vi "TagRead.vi"(7 "LabVIEW Web Service Request":refnum<class "Web Request.lvclass">, 10 "type":T1, 11 "tagName":T2) -> ()   [LabVIEW 2013]
uses:
  <vilib>/wsapi/Web Request.lvclass
  <vilib>/NI/TagWebClient/API/String Controls/tagName.ctl
  <vilib>/NI/TagWebClient/API/String Controls/type.ctl
  <vilib>/NI/Tag Bus/tag/Data Type.ctl
  <vilib>/NI/Tag Bus/table/data table.ctl
  <vilib>/NI/TagWebClient/API/JSON Formats/TagRead Response.ctl
  <vilib>/NI/TagWebClient/API/String Controls/value.ctl
  <vilib>/NI/Tag Bus/dictionary/data dictionary.lvclass
  <vilib>/NI/Tag Bus/tag/tag descriptor.lvclass
  <vilib>/NI/Tag Bus/table/data table.lvlib
  <vilib>/NI/TagWebClient/API/tagweb client API.lvlib
panel:
  out "Response String":string
  # "Use the Web Service Request input terminal to call the VIs on the Web Services palette. Do not remove it from the connector pane unless you don't need access to the palette."
  # "Each additional control wired to the connector pane will be available as an input in the URL. To include an indicator in terminal-mode output (the default setting), it must also be wired to the connector pane."
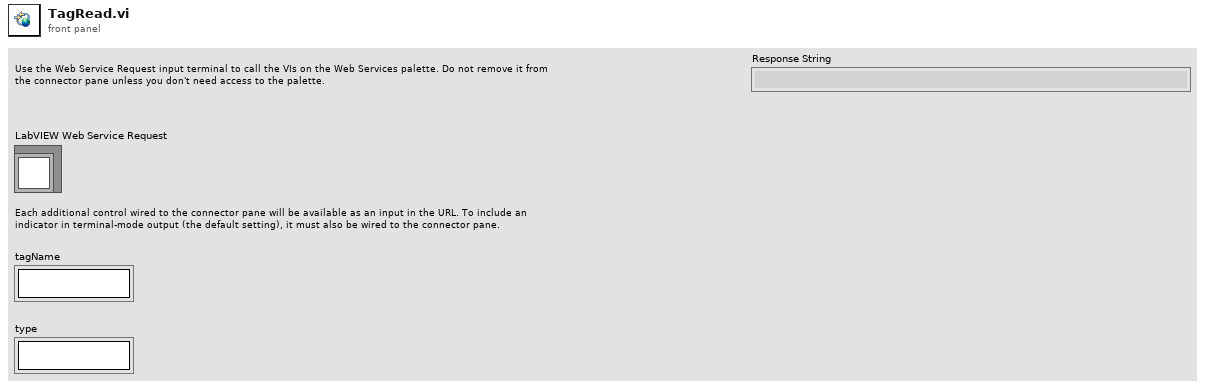
[diagram p1: front panel]
types:
  T1 = typedef "tagweb client API.lvlib/type.ctl" = string
  T2 = typedef "tagweb client API.lvlib/tagName.ctl" = string
  T3 = typedef "tag bus.lvlib/tag descriptor.lvclass/Data Type.ctl" = enum16{"Double", "Single", "I64", "I32", "I16", "I8", "U64", "U32", "U16", "U8", "Boolean", "String", "Array of Double", "Array of Single", "Array of I64", "Array of I32", "Array of I16", "Array of I8", "Array of U64", "Array of U32", "Array of U16", "Array of U8", "Array of Boolean", "Array of String"}
  T4 = typedef "tag bus.lvlib/data table.lvlib/data table.ctl" = cluster{"Double":dbl[], "Single":sgl[], "I64":i64[], "I32":i32[], "I16":i16[], "I8":i8[], "U64":u64[], "U32":u32[], "U16":u16[], "U8":u8[], "Boolean":bool[], "String":string[], "Array of Double":cluster{"DBL Array":dbl[]}[], "Array of Single":cluster{"SGL Array":sgl[]}[], "Array of I64":cluster{"I64 Array":i64[]}[], "Array of I32":cluster{"I32 Array":i32[]}[], "Array of I16":cluster{"I16 Array":i16[]}[], "Array of I8":cluster{"I8 Array":i8[]}[], "Array of U64":cluster{"U64 Array":u64[]}[], "Array of U32":cluster{"U32 Array":u32[]}[], "Array of U16":cluster{"U16 Array":u16[]}[], "Array of U8":cluster{"U8 Array":u8[]}[], "Array of Boolean":cluster{"Boolean Array":bool[]}[], "Array of String":cluster{"String Array":string[]}[]}
  T5 = typedef "tagweb client API.lvlib/TagRead Response.ctl" = cluster{"value":T6}
  T6 = typedef "tagweb client API.lvlib/value.ctl" = string
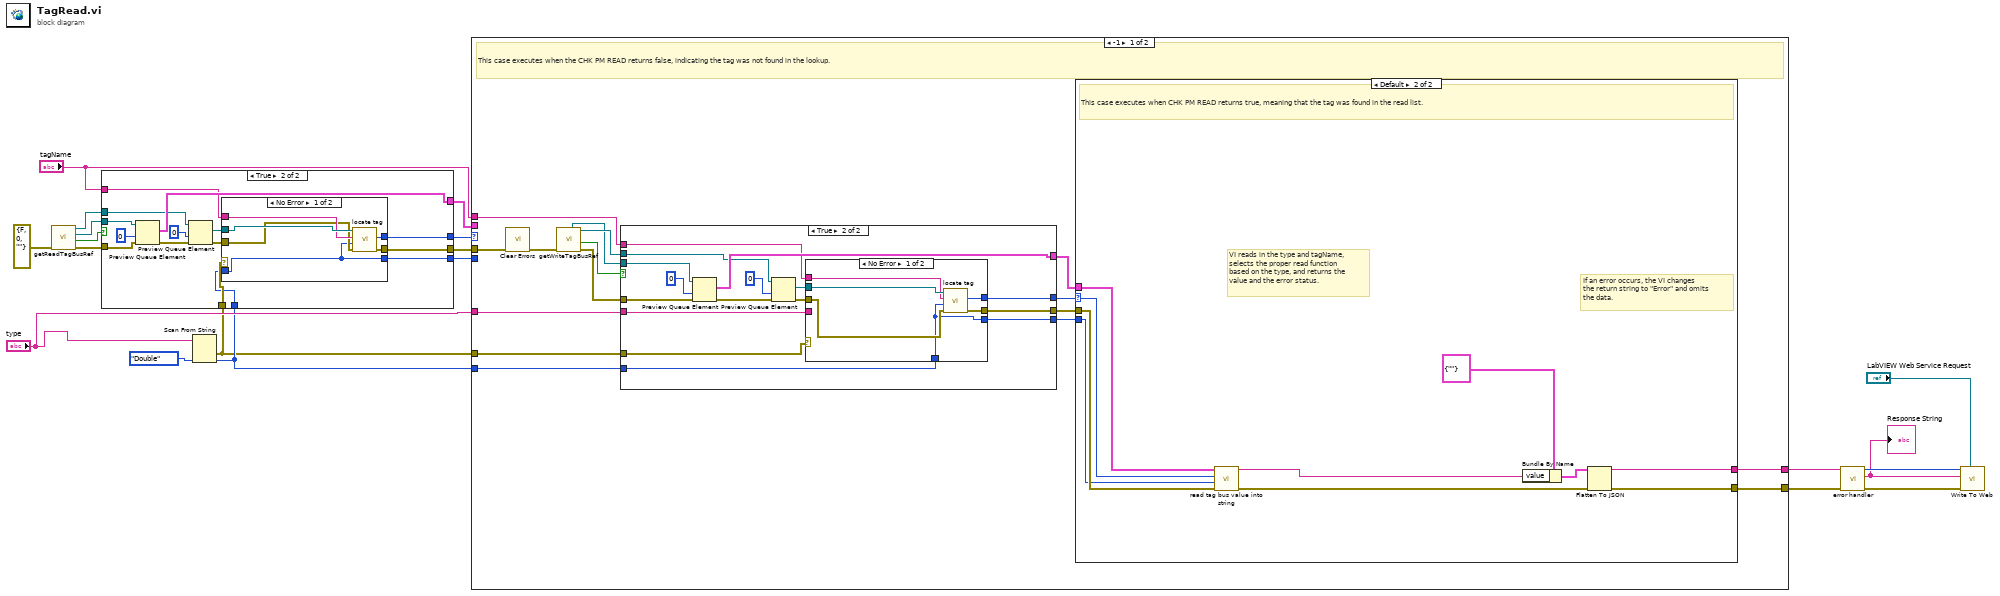
[diagram p0: block diagram]
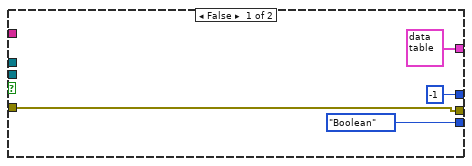
[diagram p2: hidden frame]
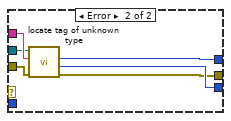
[diagram p3: hidden frame]
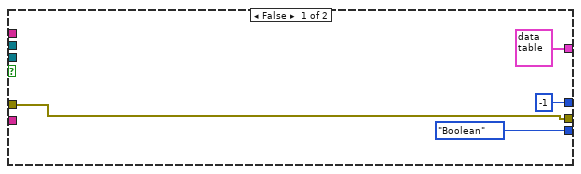
[diagram p4: hidden frame]
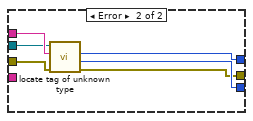
[diagram p5: hidden frame]
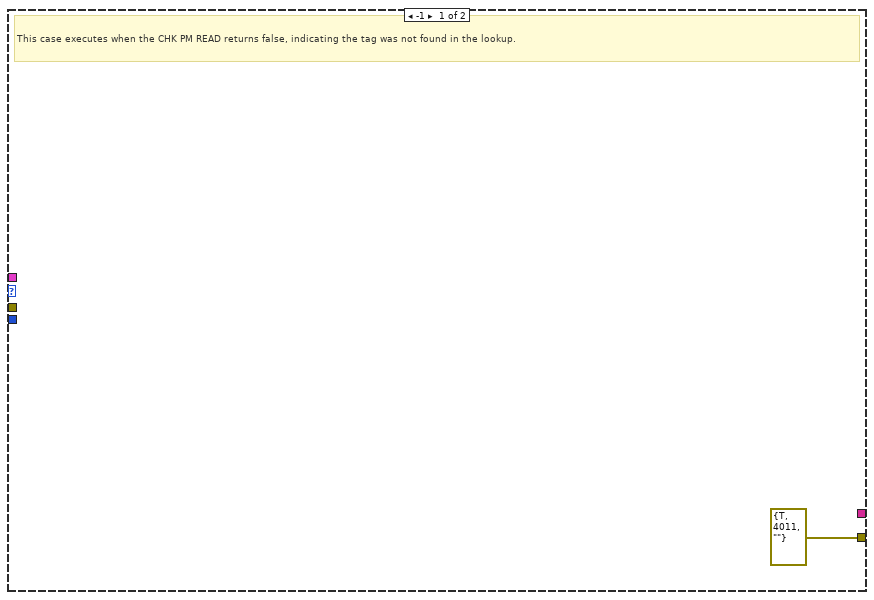
[diagram p6: hidden frame]
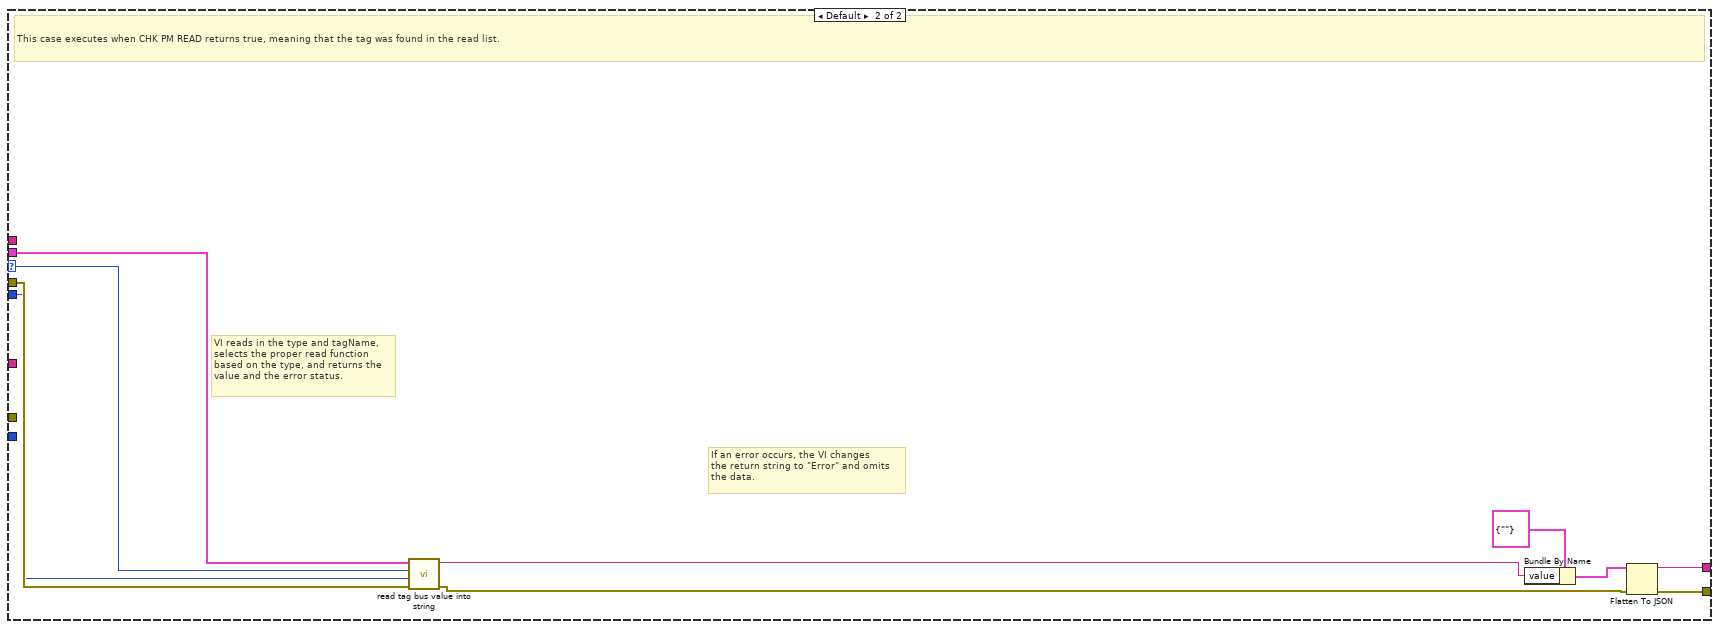
[diagram p7: hidden frame]
diagram:
  n1 = call "getReadTagBusRef.vi"("error in (no error)"=errorcluster {"status"=FALSE, "code"=0, "source"=""}) -> ("error out"=w13:errorcluster, "valid references"=w12:bool, "read data table"=w11:refnum<queue>, "read data dictionary"=w9:refnum<queue>)  [unwired: 7 in]
  n2 = Scan From String(input string="type", default 1=Data_Type."Double" ("data type")) -> (error out=w1:errorcluster, output 1=w2:T3)  [unwired: 3 in, 2 out]
  n3 = case shown="True" w12 {
    tunnel: w11 -> [_ w39]
    tunnel: [T4 {"Double"=[], "Single"=[], "I64"=[], "I32"=[], "I16"=[], "I8"=[], "U64"=[], "U32"=[], "U16"=[], "U8"=[], "Boolean"=[], "String"=[], "Array of Double"=[], "Array of Single"=[], "Array of I64"=[], "Array of I32"=[], "Array of I16"=[], "Array of I8"=[], "Array of U64"=[], "Array of U32"=[], "Array of U16"=[], "Array of U8"=[], "Array of Boolean"=[], "Array of String"=[]} ("Data Interface out") w36] -> w20
    tunnel: "tagName" -> [_ w30]
    tunnel: w13 -> [w23 w38]
    tunnel: [-1 ("index") w31] -> w18
    tunnel: [w23 w29] -> w17
    tunnel: [Data_Type."Boolean" ("data type") w32] -> w14
    tunnel: w9 -> [_ w35]
    tunnel: w1 -> [_ w26]
    tunnel: w2 -> [_ w25]
    frame False {
    }
    frame True {
      n4 = Preview Queue Element(queue=w39, timeout in ms (-1)=0, error in (no error)=w38) -> (element=w36:T4, error out=w28:errorcluster)  [unwired: 2 out]
      n5 = Preview Queue Element(queue=w35, timeout in ms (-1)=0, error in (no error)=w28) -> (element=w33:refnum<class "data dictionary.lvclass">, error out=w27:errorcluster)  [unwired: 2 out]
      n6 = case shown="No Error" w26 {
        tunnel: w33 -> [w45 w50]
        tunnel: [w40 w48] -> w32
        tunnel: [w44 w49] -> w31
        tunnel: w30 -> [w43 w51]
        tunnel: [w42 w46] -> w29
        tunnel: w27 -> [w41 w47]
        tunnel: w25 -> [w40 _]
        frame No Error {
          n7 = call <vilib>:"locate tag.vi"("error in"=w41, "data type"=w40, "name"=w43, "data dictionary in"=w45) -> ("error out"=w42:errorcluster, "index"=w44:i32)  [unwired: 5 in, 1 out]
        }
        frame Error {
          n8 = call <vilib>:"locate tag of unknown type.vi"("error in"=w47, "name"=w51, "data dictionary in"=w50) -> ("error out"=w46:errorcluster, "data type"=w48:T3, "index"=w49:i32)  [unwired: 5 in, 1 out]
        }
      }
    }
  }
  n9 = case shown="-1" w18 {
    selector: w18 -> [_ w112]
    tunnel: "tagName" -> [w64 _]
    tunnel: w17 -> [w57 w119]
    tunnel: [w58 w115] -> w16
    tunnel: [w55 w117] -> w15
    tunnel: w20 -> [_ w114]
    tunnel: w14 -> [_ w113]
    tunnel: "type" -> [w63 _]
    tunnel: w2 -> [w53 _]
    tunnel: w1 -> [w52 _]
    frame -1 {
      # "This case executes when the CHK PM READ returns false, indicating the tag was not found in the lookup."
      n10 = call <vilib>:"Clear Errors.vi"("error in (no error)"=w57) -> ("error out"=w56:errorcluster)  [unwired: 6 in]
      n11 = call "getWriteTagBusRef.vi"("error in"=w56) -> ("error out"=w65:errorcluster, "valid references"=w66:bool, "write data dictionary"=w67:refnum<queue>, "actual write data table"=w54:refnum<queue>)  [unwired: 6 in, 1 out]
      n12 = case shown="True" w66 {
        tunnel: w54 -> [_ w87]
        tunnel: [T4 {"Double"=[], "Single"=[], "I64"=[], "I32"=[], "I16"=[], "I8"=[], "U64"=[], "U32"=[], "U16"=[], "U8"=[], "Boolean"=[], "String"=[], "Array of Double"=[], "Array of Single"=[], "Array of I64"=[], "Array of I32"=[], "Array of I16"=[], "Array of I8"=[], "Array of U64"=[], "Array of U32"=[], "Array of U16"=[], "Array of U8"=[], "Array of Boolean"=[], "Array of String"=[]} ("Data Interface out") w84] -> w61
        tunnel: w64 -> [_ w77]
        tunnel: w65 -> [w70 w86]
        tunnel: [-1 ("index") w78] -> w60
        tunnel: [w70 w76] -> w59
        tunnel: [Data_Type."Boolean" ("data type") w79] -> w62
        tunnel: w67 -> [_ w83]
        tunnel: w63 -> [_ w81]
        tunnel: w53 -> [_ w73]
        tunnel: w52 -> [_ w72]
        frame False {
        }
        frame True {
          n13 = Preview Queue Element(queue=w87, timeout in ms (-1)=0, error in (no error)=w86) -> (element=w84:T4, error out=w75:errorcluster)  [unwired: 2 out]
          n14 = Preview Queue Element(queue=w83, timeout in ms (-1)=0, error in (no error)=w75) -> (element=w80:refnum<class "data dictionary.lvclass">, error out=w74:errorcluster)  [unwired: 2 out]
          n15 = case shown="No Error" w72 {
            tunnel: w81 -> [_ _]
            tunnel: w80 -> [w93 w98]
            tunnel: [w88 w96] -> w79
            tunnel: [w92 w97] -> w78
            tunnel: w77 -> [w91 w99]
            tunnel: [w90 w94] -> w76
            tunnel: w74 -> [w89 w95]
            tunnel: w73 -> [w88 _]
            frame No Error {
              n16 = call <vilib>:"locate tag.vi"("error in"=w89, "data type"=w88, "name"=w91, "data dictionary in"=w93) -> ("error out"=w90:errorcluster, "index"=w92:i32)  [unwired: 5 in, 1 out]
            }
            frame Error {
              n17 = call <vilib>:"locate tag of unknown type.vi"("error in"=w95, "name"=w99, "data dictionary in"=w98) -> ("error out"=w94:errorcluster, "data type"=w96:T3, "index"=w97:i32)  [unwired: 5 in, 1 out]
            }
          }
        }
      }
      n18 = case shown="Default" w60 {
        selector: w60 -> [_ w101]
        tunnel: w59 -> [_ w106]
        tunnel: [errorcluster {"status"=TRUE, "code"=4011, "source"=""} ("error in (no error)") w108] -> w58
        tunnel: [_ w109] -> w55
        tunnel: w61 -> [_ w103]
        tunnel: w62 -> [_ w102]
        frame -1 {
          # "This case executes when the CHK PM READ returns false, indicating the tag was not found in the lookup."
        }
        frame Default {
          # "If an error occurs, the VI changes\nthe return string to \"Error\" and omits\nthe data."
          # "VI reads in the type and tagName,\nselects the proper read function\nbased on the type, and returns the\nvalue and the error status."
          # "This case executes when CHK PM READ returns true, meaning that the tag was found in the read list."
          n19 = call "read tag bus value into string.vi"("error in (no error)"=w106, "data type"=w102, "index"=w101, "data table"=w103) -> ("error out"=w105:errorcluster, "Value"=w104:string)  [unwired: 6 in]
          n20 = Bundle By Name(cluster=T5 {"value"=""}, "value"=w104) -> (w110:T5)
          n21 = Flatten To JSON(anything=w110, error in (no error)=w105) -> (JSON string=w109:string, 11:w108:errorcluster)  [unwired: 1 in]
        }
      }
    }
    frame Default {
      # "If an error occurs, the VI changes\nthe return string to \"Error\" and omits\nthe data."
      # "VI reads in the type and tagName,\nselects the proper read function\nbased on the type, and returns the\nvalue and the error status."
      # "This case executes when CHK PM READ returns true, meaning that the tag was found in the read list."
      n22 = call "read tag bus value into string.vi"("error in (no error)"=w119, "data type"=w113, "index"=w112, "data table"=w114) -> ("error out"=w116:errorcluster, "Value"=w120:string)  [unwired: 6 in]
      n23 = Bundle By Name(cluster=T5 {"value"=""}, "value"=w120) -> (w118:T5)
      n24 = Flatten To JSON(anything=w118, error in (no error)=w116) -> (JSON string=w117:string, 11:w115:errorcluster)  [unwired: 1 in]
    }
  }
  n25 = call "error handler.vi"("error in (no error)"=w16, "Success Message"=w15) -> ("error out"=w8:errorcluster, "Response String"=w5:string, "Response Code"=w6:i32)  [unwired: 7 in]
  "Response String" <- w5
  n26 = call <vilib>:"Write To Web.vi"("Web Request in"="LabVIEW Web Service Request", "error in (no error)"=w8, "Response String"=w5, "Response Code"=w6) -> ()  [unwired: 7 in, 1 out]
